vi "TiePie.Lst.LstDevCanOpen.vi"(8 "error in (no error)":errorcluster, 9 "dwDeviceType":u32, 10 "dwId":u32, 11 "dwIdKind":u32) -> (0 "error out":errorcluster, 2 "return type":u8)   [LabVIEW 2014, in "LVTiePie.lvlib"]
uses:
  LVTiePie.lvlib
  bin/libtiepie.dll
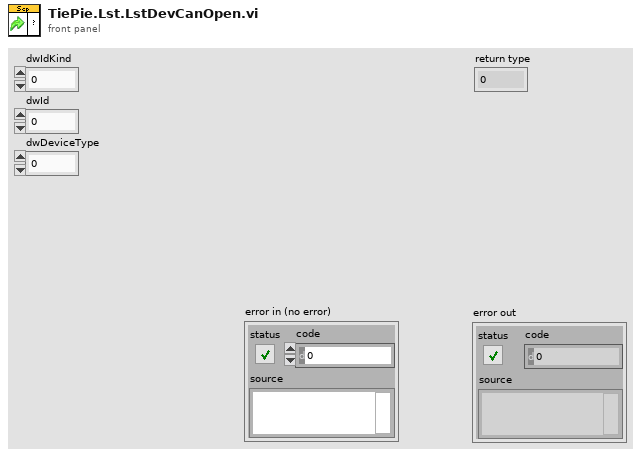
[diagram p1: front panel]
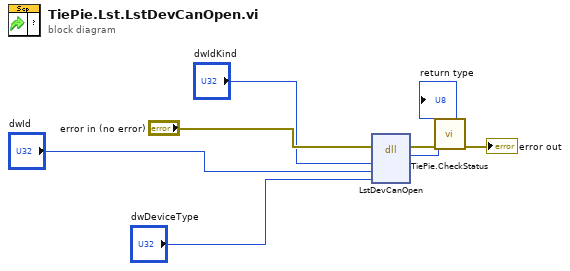
[diagram p0: block diagram]
diagram:
  n1 = dll-call lib="C:/Users/mbirski/Desktop/PAN/LabVEW/Tie Pie/bin/libtiepie.dll" fn="LstDevCanOpen"(error in="error in (no error)", "dwIdKind"="dwIdKind", "dwId"="dwId", "dwDeviceType"="dwDeviceType") -> (error out=w6:errorcluster, "canBeOpened"=→"return type":u8)  [unwired: 5 in, 1 out]
  n2 = call "TiePie.CheckStatus.vi"("error in (no error)"=w6) -> ("error out"=→"error out":errorcluster)  [unwired: 10 in]
